vi "belezenje.vi"() -> ()   [LabVIEW 2021]
panel:
  in  "zaporedni_set":dbl
  out "ID":dbl
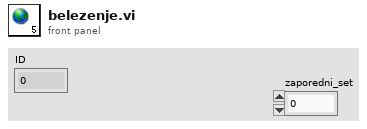
[diagram p1: front panel]
diagram:
